vi "adresse.vi"() -> ()   [LabVIEW 2019]
uses:
  <vilib>/rvi/eio/common/nirviEmuTemplateMethod_errors.vi
  <vilib>/eio/EIONode/EIONode.xnode
panel:
  in  "Address WHO I AM register":bool[](array[boolean])
  in  "Read(1)/Write(0)":bool
  in  "Address accelerator sensor":bool[](array[boolean])
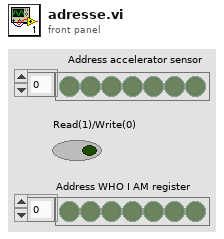
[diagram p1: front panel]
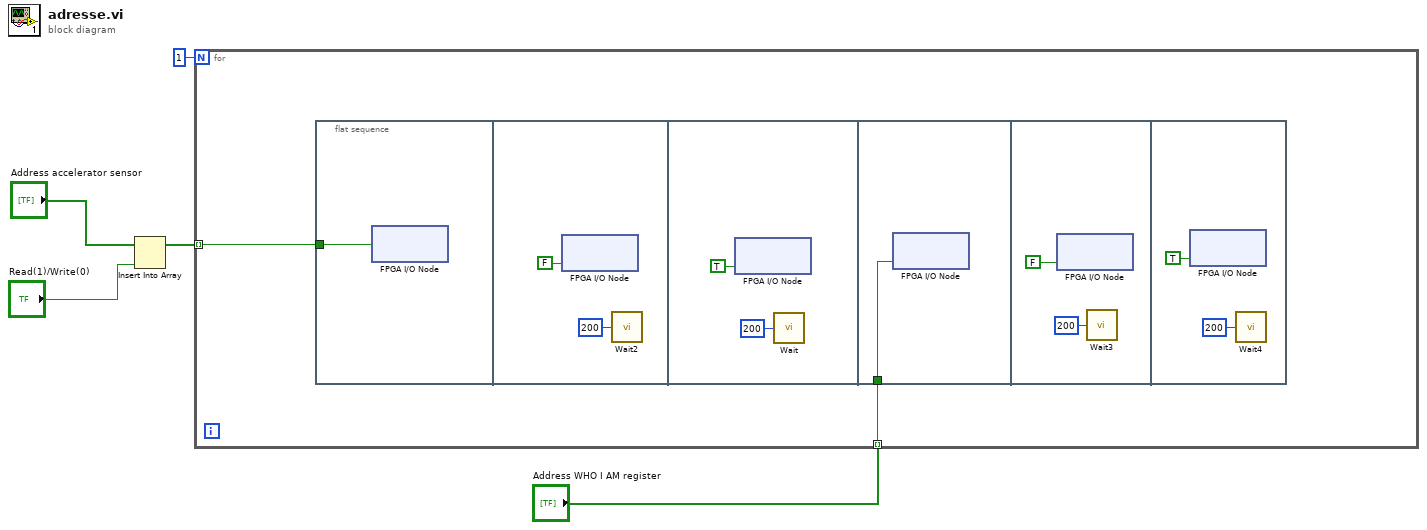
[diagram p0: block diagram]
diagram:
  n1 = Insert Into Array(array="Address accelerator sensor", new element="Read(1)/Write(0)") -> (w3:bool[])  [unwired: 1 in]
  n2 = for {
    N: 1 -> [_]
    tunnel: w3 -> [w7] mode=indexing
    tunnel: "Address WHO I AM register" -> [w6] mode=indexing
    n3 = flat-sequence {
      tunnel: w7 -> [w8]
      tunnel: w6 -> [w13]
      frame #0 {
        n4 = xnode "FPGA I/O Node"("SDA"=w8) -> ()  [unwired: 1 in, 1 out]
      }
      frame #1 {
        n5 = xnode "FPGA I/O Node"("SCL"=FALSE) -> ()  [unwired: 1 in, 1 out]
        n6 = call "Wait2"("Count(Ticks)"=u32 200) -> ()  [unwired: 1 out]
      }
      frame #2 {
        n7 = xnode "FPGA I/O Node"("SCL"=TRUE) -> ()  [unwired: 1 in, 1 out]
        n8 = call "Wait"("Count(Ticks)"=u32 200) -> ()  [unwired: 1 out]
      }
      frame #3 {
        n9 = xnode "FPGA I/O Node"("SDA"=w13) -> ()  [unwired: 1 in, 1 out]
      }
      frame #4 {
        n10 = xnode "FPGA I/O Node"("SCL"=FALSE) -> ()  [unwired: 1 in, 1 out]
        n11 = call "Wait3"("Count(Ticks)"=u32 200) -> ()  [unwired: 1 out]
      }
      frame #5 {
        n12 = xnode "FPGA I/O Node"("SCL"=TRUE) -> ()  [unwired: 1 in, 1 out]
        n13 = call "Wait4"("Count(Ticks)"=u32 200) -> ()  [unwired: 1 out]
      }
    }
  }
